vi "AfterPage2_UI.vi"(10 "MetaDataObj":refnum<class "MetaDataObj.lvclass">) -> ()   [LabVIEW 2021, in "Plugin_Generator.lvclass"]
uses:
  Plugin_Generator.lvclass
  <resource>/dialog/NewProjectWizard/MetaDataObj/MetaDataObj.lvclass
  CIF-LVCore/src/Channels/ChannelRegistrar/typedef/Channel Definition for Scripting.ctl
  <vilib>/CIF Foundation/CIF Channels Core/CIFChannels/Typedef/Direction.ctl
  CIF-LVCore/src/Channels/ChannelRegistrar/typedef/Registered Channel Types.ctl
  C:/Program Files/National Instruments/LabVIEW 2021/resource/dialog/NewProjectWizard/MetaDataObj/MetaDataObj.lvclass
  Plugin_Generator.lvclass/Plugin_Generator.ctl
  <resource>/dialog/NewProjectWizard/MetaDataObj/MetaDataObj.lvclass/MetaDataObj.ctl
  <resource>/dialog/NewProjectWizard/MetaDataObj/Accessors/Read Project Name.vi
  <resource>/dialog/NewProjectWizard/MetaDataObj/Accessors/Read Project Root.vi
  <resource>/dialog/NewProjectWizard/Project Copying/NI_NPW_Project Copying.lvlib
  <vilib>/CIF Foundation/CIF Channels Core/CIFChannels/CIFChannels.lvclass
  CIF-LVCore/src/Channels/ChannelRegistrar/ChannelRegistrar.lvlib
panel:
  out "Channels to Create":T1[](array[typedef])
  out "Project Root":path
  out "Project Name":string
  out "Payload Name":string
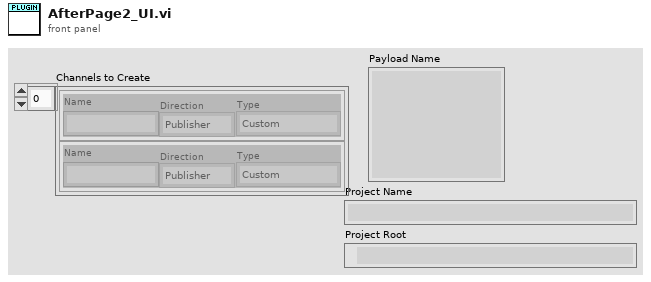
[diagram p1: front panel]
types:
  T1 = typedef "ChannelRegistrar.lvlib/Channel Definition for Scripting.ctl" = cluster{"Name":string, "Direction":T2, "Type":T3}
  T2 = typedef "CIFChannels.lvclass/Direction.ctl" = enum16{"Publisher", "Subscriber"}
  T3 = typedef "ChannelRegistrar.lvlib/Registered Channel Types.ctl" = enum16{"Custom", "Double_Tag", "I64_Tag", "U64_Tag", "U8_FIFO", "CAN_FIFO", "L2Enet_FIFO", "DAQ_FIFO", "Universal_FIFO", "String_Tag"}
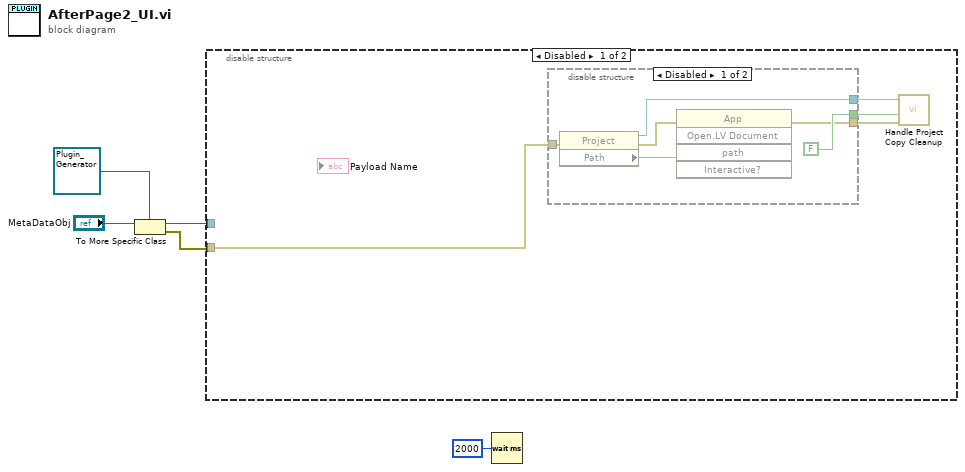
[diagram p0: block diagram]
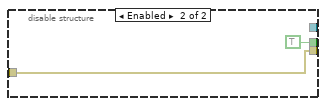
[diagram p2: hidden frame]
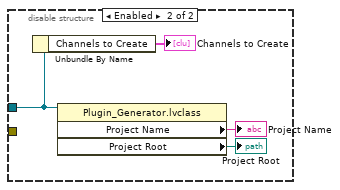
[diagram p3: hidden frame]
diagram:
  n1 = To More Specific Class(target class=refnum<class "Plugin_Generator.lvclass"> refnum ("Plugin_Generator.lvclass"), reference="MetaDataObj") -> (specific class reference=w3:refnum<class "Plugin_Generator.lvclass">, error out=w2:errorcluster)  [unwired: 1 in]
  n2 = disable-structure shown="Disabled" {
    disable-tunnel: w2 -> [w6 _]
    disable-tunnel: w3 -> [_ w19]
    frame Disabled {
      n3 = disable-structure shown="Disabled" {
        disable-tunnel: w6 -> [w13 w17]
        disable-tunnel: [FALSE ("More Scripting?") TRUE ("More Scripting?")] -> w9
        disable-tunnel: [w11 w17] -> w8
        disable-tunnel: [w10 _] -> w7
        frame Disabled {
          n4 = property class="Project"(error in=w13) -> (reference out=w10:refnum<vi>, error out=w14:errorcluster, "Path"=w15:path)  [unwired: 1 in]
          n5 = invoke class="App" method="Open.LV Document"(error in=w14, "path"=w15) -> (error out=w11:errorcluster)  [unwired: 3 in, 4 out]
        }
        frame Enabled {
        }
      }
      n6 = call <resource>:"Handle Project Copy Cleanup.vi"("error in (no error)"=w8, "More Scripting?"=w9, "Project in"=w7) -> ()  [unwired: 9 in]
    }
    frame Enabled {
      n7 = Unbundle By Name(w19) -> ("Channels to Create"=→"Channels to Create":T1[])
      n8 = property class="Plugin_Generator.lvclass"(reference=w19) -> ("Project Name"=→"Project Name":string, "Project Root"=→"Project Root":path)  [unwired: 1 in, 2 out]
    }
  }
  n9 = Wait (ms)(milliseconds to wait=u32 2000) -> ()  [unwired: 1 out]
